vi "threshConvert.vi"(10 "error in":errorcluster, 11 "Select Threshold Value":u16) -> (2 "error out":errorcluster, 3 "Threshold Frame":string)   [LabVIEW 2018]
panel:
  out "hex integer string":string
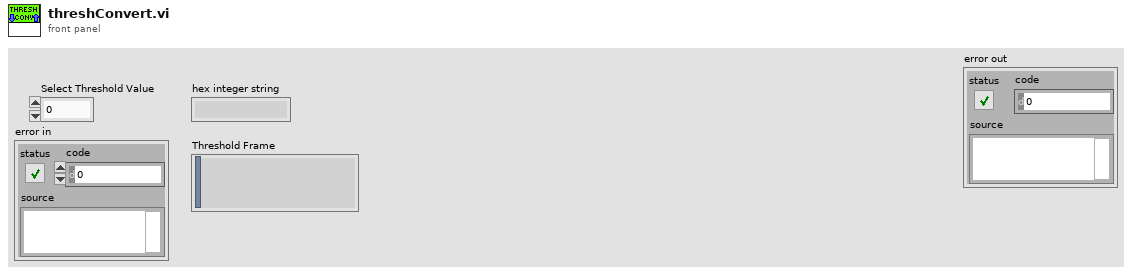
[diagram p1: front panel]
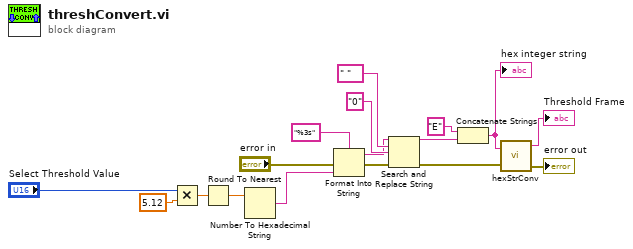
[diagram p0: block diagram]
diagram:
  n1 = Multiply(x="Select Threshold Value", y=5.12) -> (x*y=w4:dbl)
  n2 = Round To Nearest(number=w4) -> (nearest integer value=w5:dbl)
  n3 = Number To Hexadecimal String(2:w5) -> (0:w8:string)  [unwired: 1 in]
  n4 = Format Into String(format string="%3s", error in="error in", w8) -> (resulting string=w6:string, error out=w16:errorcluster)  [unwired: 1 in]
  n5 = Search and Replace String(input string=w6, search string=" ", replace string="0" ("replace string (\"\")"), error in=w16) -> (result string=w12:string, error out=w15:errorcluster)  [unwired: 4 in, 2 out]
  n6 = Concatenate Strings("E", w12) -> (w13:string)
  "hex integer string" <- w13
  n7 = call "hexStrConv.vi"("Input ASCII Hex String"=w13, "error in (no error)"=w15) -> ("Output Non Printable HEX String"=→"Threshold Frame":string, "error out"=→"error out":errorcluster)  [unwired: 1 out]
